vi "Scan Path Folder.vi"(6 "error in":errorcluster, 7 "Current Depth":dbl, 8 "Max Depth":dbl, 9 "Parent Tag":string, 11 "Path":path) -> (2 "File Items":T1(array[cluster]), 3 "Folder Items":T1(array[cluster]))   [LabVIEW 2025]
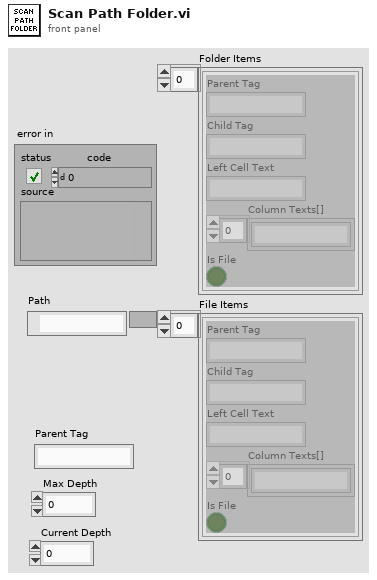
[diagram p1: front panel]
types:
  T1 = cluster{"Parent Tag":string, "Child Tag":string, "Left Cell Text":string, "Column Texts[]":string[], "Is File":bool}[]
  T2 = cluster{"Parent Tag":string, "Child Tag":string, "Left Cell Text":string, "Column Texts[]":string[], "Is File":bool}
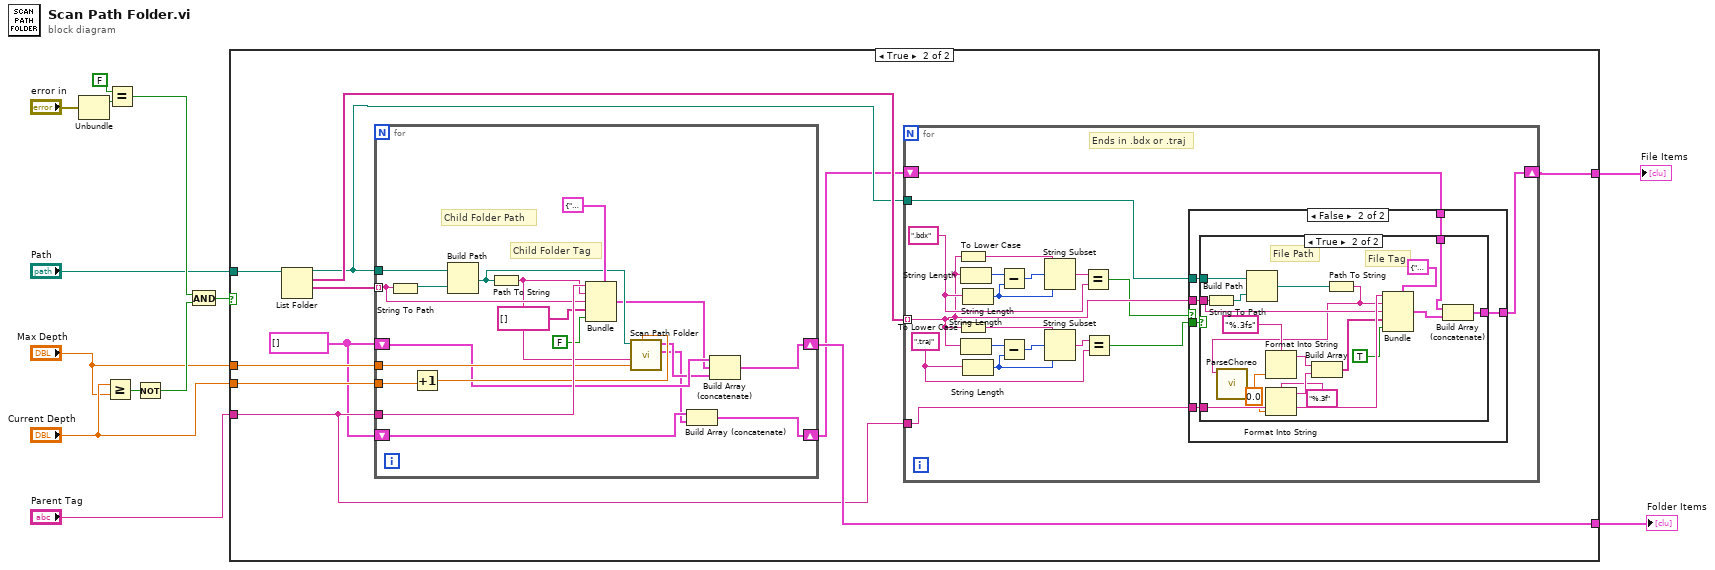
[diagram p0: block diagram]
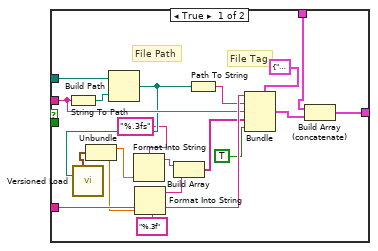
[diagram p3: hidden frame]
diagram:
  n1 = Unbundle("error in") -> ("status"=w12:bool)  [unwired: 2 out]
  n2 = Greater Or Equal?(x="Current Depth", y="Max Depth") -> (x >= y?=w7:bool)
  n3 = Equal?(x=FALSE, y=w12) -> (x = y?=w9:bool)
  n4 = Not(x=w7) -> (.not. x?=w8:bool)
  n5 = And(x=w9, y=w8) -> (x .and. y?=w10:bool)
  n6 = case shown="True" w10 {
    tunnel: "Path" -> [_ w24]
    tunnel: "Parent Tag" -> [_ w17]
    tunnel: "Current Depth" -> [_ w22]
    tunnel: "Max Depth" -> [_ w21]
    tunnel: [_ w20] -> w2
    tunnel: [_ w16] -> w1
    frame False {
    }
    frame True {
      w15 = T1 []
      n7 = List Folder(path=w24) -> (path out=w18:path, filenames=w19:string[], folder names=w23:string[])  [unwired: 3 in, 1 out]
      n8 = for {
        tunnel: w23 -> [w103] mode=indexing
        tunnel: w18 -> [w106]
        tunnel: w17 -> [w104]
        tunnel: w22 -> [w97]
        tunnel: w21 -> [w95]
        shift-right: [w92] -> w20
        shift-left: w15 -> [w94]
        shift-right: [w88] -> w14
        shift-left: w15 -> [w90]
        # "Child Folder Tag"
        # "Child Folder Path"
        n9 = String To Path(string=w103) -> (path=w105:path)
        n10 = Increment(x=w97) -> (x+1=w96:dbl)
        n11 = Build Path(base path=w106, name or relative path=w105) -> (appended path=w99:path)
        n12 = Path To String(path=w99) -> (string=w98:string)
        n13 = Bundle(cluster=T2 {"Parent Tag"="", "Child Tag"="", "Left Cell Text"="", "Column Texts[]"=[], "Is File"=FALSE} ("Tree Item 2"), "Parent Tag"=w104, "Child Tag"=w98, "Left Cell Text"=w103, "Column Texts[]"=string[] [], "Is File"=FALSE) -> (w93:T2)
        n14 = call "Scan Path Folder.vi"("Current Depth"=w96, "Max Depth"=w95, "Parent Tag"=w98, "Path"=w99) -> ("File Items"=w89:T1, "Folder Items"=w91:T1)  [unwired: 6 in]
        n15 = Build Array (concatenate)(w90, w89) -> (w88:T1)
        n16 = Build Array (concatenate)(w94, w93, w91) -> (w92:T1)
      }
      n17 = for {
        tunnel: w19 -> [w30] mode=indexing
        tunnel: w18 -> [w31]
        tunnel: w17 -> [w29]
        shift-right: [w27] -> w16
        shift-left: w14 -> [w28]
        w33 = ".traj" ("string")
        w32 = ".bdx"
        # "Ends in .bdx or .traj"
        n18 = To Lower Case(string=w30) -> (all lower case string=w43:string)
        n19 = To Lower Case(string=w30) -> (all lower case string=w38:string)
        n20 = String Length(string=w30) -> (length=w42:i32)
        n21 = String Length(string=w30) -> (length=w37:i32)
        n22 = String Length(string=w32) -> (length=w41:i32)
        n23 = String Length(string=w33) -> (length=w36:i32)
        n24 = Subtract(x=w42, y=w41) -> (x-y=w40:i32)
        n25 = Subtract(x=w37, y=w36) -> (x-y=w35:i32)
        n26 = String Subset(string=w43, offset (0)=w40, length (rest)=w41) -> (substring=w39:string)
        n27 = String Subset(string=w38, offset (0)=w35, length (rest)=w36) -> (substring=w34:string)
        n28 = Equal?(x=w39, y=w32) -> (x = y?=w26:bool)
        n29 = Equal?(x=w34, y=w33) -> (x = y?=w25:bool)
        n30 = case shown="False" w26 {
          tunnel: w31 -> [w62 w68]
          tunnel: w30 -> [w58 w66]
          tunnel: w29 -> [w60 w67]
          tunnel: w28 -> [w55 w65]
          tunnel: [w53 w64] -> w27
          tunnel: w25 -> [_ w63]
          frame True {
            # "File Tag"
            # "File Path"
            n31 = String To Path(string=w58) -> (path=w61:path)
            n32 = Build Path(base path=w62, name or relative path=w61) -> (appended path=w51:path)
            n33 = call "Versioned Load.vi"("path"=w51) -> ("Overall"=w52:cluster{"Time (s)":dbl, "Distance (ft)":dbl})  [unwired: 6 in, 8 out]
            n34 = Unbundle(w52) -> ("Time (s)"=w49:dbl, "Distance (ft)"=w48:dbl)
            n35 = Format Into String(format string="%.3fs", w49) -> (resulting string=w47:string)  [unwired: 2 in, 1 out]
            n36 = Format Into String(format string="%.3f", w48) -> (resulting string=w46:string)  [unwired: 2 in, 1 out]
            n37 = Build Array(w47, w46) -> (w50:string[])
            n38 = Path To String(path=w51) -> (string=w59:string)
            n39 = Bundle(cluster=T2 {"Parent Tag"="", "Child Tag"="", "Left Cell Text"="", "Column Texts[]"=[], "Is File"=FALSE} ("Tree Item 2"), "Parent Tag"=w60, "Child Tag"=w59, "Left Cell Text"=w58, "Column Texts[]"=w50, "Is File"=TRUE) -> (w54:T2)
            n40 = Build Array (concatenate)(w55, w54) -> (w53:T1)
          }
          frame False {
            n41 = case shown="True" w63 {
              tunnel: w68 -> [_ w87]
              tunnel: w67 -> [_ w84]
              tunnel: w66 -> [_ w83]
              tunnel: w65 -> [w69 w80]
              tunnel: [w69 w78] -> w64
              frame False {
              }
              frame True {
                # "File Tag"
                # "File Path"
                n42 = String To Path(string=w83) -> (path=w86:path)
                n43 = Build Path(base path=w87, name or relative path=w86) -> (appended path=w85:path)
                n44 = Format Into String(format string="%.3f", 0.0 ("input 1")) -> (resulting string=w74:string)  [unwired: 2 in, 1 out]
                n45 = Path To String(path=w85) -> (string=w72:string)
                n46 = call "ParseChoreo.vi"("FileName"=w72) -> ("TrajTime"=w71:dbl)  [unwired: 6 in, 4 out]
                n47 = Format Into String(format string="%.3fs", w71) -> (resulting string=w75:string)  [unwired: 2 in, 1 out]
                n48 = Build Array(w75, w74) -> (w77:string[])
                n49 = Bundle(cluster=T2 {"Parent Tag"="", "Child Tag"="", "Left Cell Text"="", "Column Texts[]"=[], "Is File"=FALSE} ("Tree Item 2"), "Parent Tag"=w84, "Child Tag"=w72, "Left Cell Text"=w83, "Column Texts[]"=w77, "Is File"=TRUE) -> (w79:T2)
                n50 = Build Array (concatenate)(w80, w79) -> (w78:T1)
              }
            }
          }
        }
      }
    }
  }
  "Folder Items" <- w2
  "File Items" <- w1
